vi "CircularLoop.vi"() -> ()   [LabVIEW 2018]
panel:
  out "Intensity Chart":dbl[][](graph)
  out "yEndpoints":dbl[](array[numeric])
  out "xEndpoints":dbl[](array[numeric])
  in  "current":dbl
  in  "radius":dbl
  in  "sides":dbl
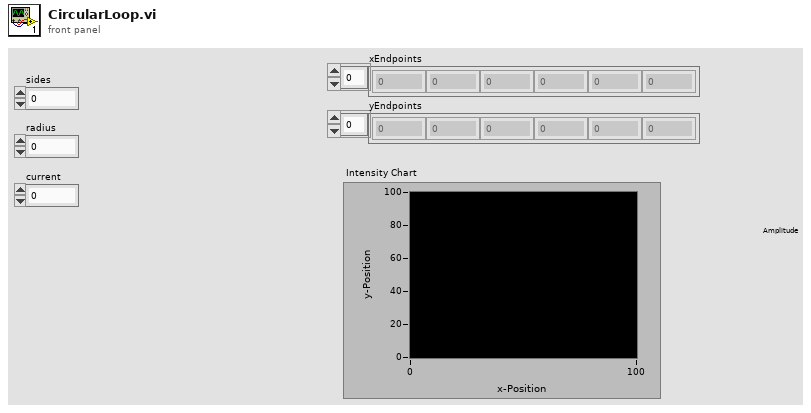
[diagram p1: front panel]
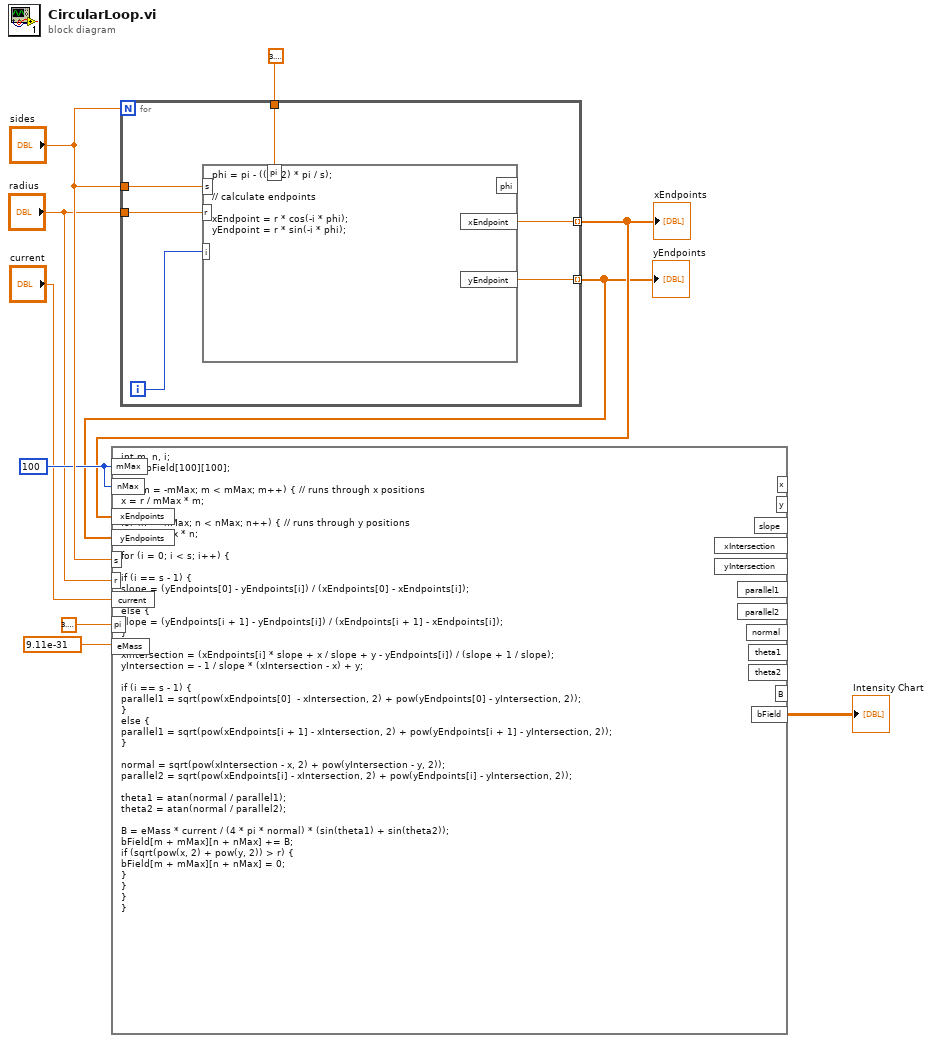
[diagram p0: block diagram]
diagram:
  w8 = 100
  n1 = for {
    N: "sides" -> [_]
    tunnel: "sides" -> [w16]
    tunnel: 3.141592653589793 -> [w15]
    tunnel: "radius" -> [w13]
    tunnel: [w12] -> w7 mode=indexing
    tunnel: [w11] -> w6 mode=indexing
    i -> [w14]
    n2 = formula code="phi = pi - ((s - 2) * pi / s);\n\n// calculate endpoints\n\nxEndpoint = r * cos(-i * phi);\nyEndpoint = r * sin(-i * phi);"("s"=w16, "pi"=w15, "i"=w14, "r"=w13) -> ("xEndpoint"=w12:dbl, "yEndpoint"=w11:dbl)  [unwired: 1 out]
  }
  "xEndpoints" <- w7
  "yEndpoints" <- w6
  n3 = formula code="int m, n, i;\nfloat bField[100][100];\n\nfor (m = -mMax; m < mMax; m++) { // runs through x positions\nx = r / mMax * m;\n\nfor (n = -nMax; n < nMax; n++) { // runs through y positions\ny = r / nMax * n;\n\nfor (i = 0; i < s; i++) {\n\nif (i == s - 1) {\nslope = (yEndpoints[0] - yEndpoints[i]) / (xEndpoints[0] - xEndpoints[i]);\n}\nelse {\nslope = (yEndpoints[i + 1] - yEndpoints[i]) / (xEndpoints[i + 1] - xEndpoints[i]);\n}\n\nxIntersection = (xEndpoints[i] * slope + x / slope + y - yEndpoints[i]) / (slope + 1 / slope);\nyIntersection = - 1 / slope * (xIntersection - x) + y;\n\nif (i == s - 1) {\nparallel1 = sqrt(pow(xEndpoints[0]  - xIntersection, 2) + pow(yEndpoints[0] - yIntersection, 2));  \n}\nelse {\nparallel1 = sqrt(pow(xEndpoints[i + 1] - xIntersection, 2) + pow(yEndpoints[i + 1] - yIntersection, 2));\n}\n\nnormal = sqrt(pow(xIntersection - x, 2) + pow(yIntersection - y, 2));\nparallel2 = sqrt(pow(xEndpoints[i] - xIntersection, 2) + pow(yEndpoints[i] - yIntersection, 2));\n\ntheta1 = atan(normal / parallel1);\ntheta2 = atan(normal / parallel2);\n\nB = eMass * current / (4 * pi * normal) * (sin(theta1) + sin(theta2));\nbField[m + mMax][n + nMax] += B;\nif (sqrt(pow(x, 2) + pow(y, 2)) > r) {\nbField[m + mMax][n + nMax] = 0;\n}\n}\n}\n}"("mMax"=w8, "s"="sides", "nMax"=w8, "xEndpoints"=w7, "yEndpoints"=w6, "r"="radius", "current"="current", "pi"=3.141592653589793, "eMass"=9.11e-31) -> ("bField"=→"Intensity Chart":dbl[][])  [unwired: 11 out]
